vi "Analy Json.vi"(8 "error in (no error)":errorcluster, 10 "body":string="{\"error_code\":0,\"error_msg\":\"SUCCESS\",\"log_id\":3501517038,\"timestamp\":1684306701,\"cached\":0,\"result\":{\"face_num\":7,\"face_list\":[{\"face_token\":\"9dc85bb57dba77ceee2717260b4e6c8a\",\"location\":{\"left\":515.27,\"top\":41.56,\"width\":29,\"height\":31,\"rotation\":13},\"face_probability\":1,\"angle\":{\"yaw\":21.28,\"pitch\":5.54,\"roll\":10.68}},{\"face_token\":\"519822cd005f9fd56a774038260bf9c1\",\"location\":{\"left\":242.84,\"top\":19.73,\"width\":29,\"height\":29,\"rotation\":33},\"face_probability\":1,\"angle\":{\"yaw\":-2.53,\"pitch\":12.63,\"roll\":30.73}},{\"face_token\":\"0cb54c44f353f8f4b24468424f908c8a\",\"location\":{\"left\":150.92,\"top\":30.76,\"width\":30,\"height\":28,\"rotation\":6},\"face_probability\":0.99,\"angle\":{\"yaw\":-1.15,\"pitch\":9.32,\"roll\":2.81}},{\"face_token\":\"8612e393bdc06ac7a96a46a15dd12818\",\"location\":{\"left\":367.55,\"top\":29.17,\"width\":27,\"height\":31,\"rotation\":9},\"face_probability\":1,\"angle\":{\"yaw\":-14.5,\"pitch\":3.18,\"roll\":7.23}},{\"face_token\":\"1f123ecde6098c6bc67fbb6ddb0b806a\",\"location\":{\"left\":447,\"top\":38.09,\"width\":29,\"height\":27,\"rotation\":10},\"face_probability\":1,\"angle\":{\"yaw\":-8.18,\"pitch\":8.23,\"roll\":10.84}},{\"face_token\":\"b994523fe7b95fddfed7fbed407f0b6f\",\"location\":{\"left\":80.83,\"top\":43.37,\"width\":30,\"height\":26,\"rotation\":23},\"face_probability\":1,\"angle\":{\"yaw\":-14.98,\"pitch\":12.31,\"roll\":24.44}},{\"face_token\":\"da3ec671683a7d13f9daffcd54db10f0\",\"location\":{\"left\":300.6,\"top\":29.25,\"width\":28,\"height\":27,\"rotation\":9},\"face_probability\":1,\"angle\":{\"yaw\":-7.29,\"pitch\":8.2,\"roll\":7.41}}]}}" caption="体部") -> (0 "error out":errorcluster, 2 "face_list":T3[](array[typedef]), 3 "All info":T1)   [LabVIEW 2025]
uses:
  controls/face_list.ctl
  controls/All info.ctl
  controls/Return Info.ctl
  <vilib>/addons/_JKI.lib/Serialization/JSON/JKI JSON Serialization.lvlib
  <vilib>/Utility/Data Type/NI_Data Type.lvlib
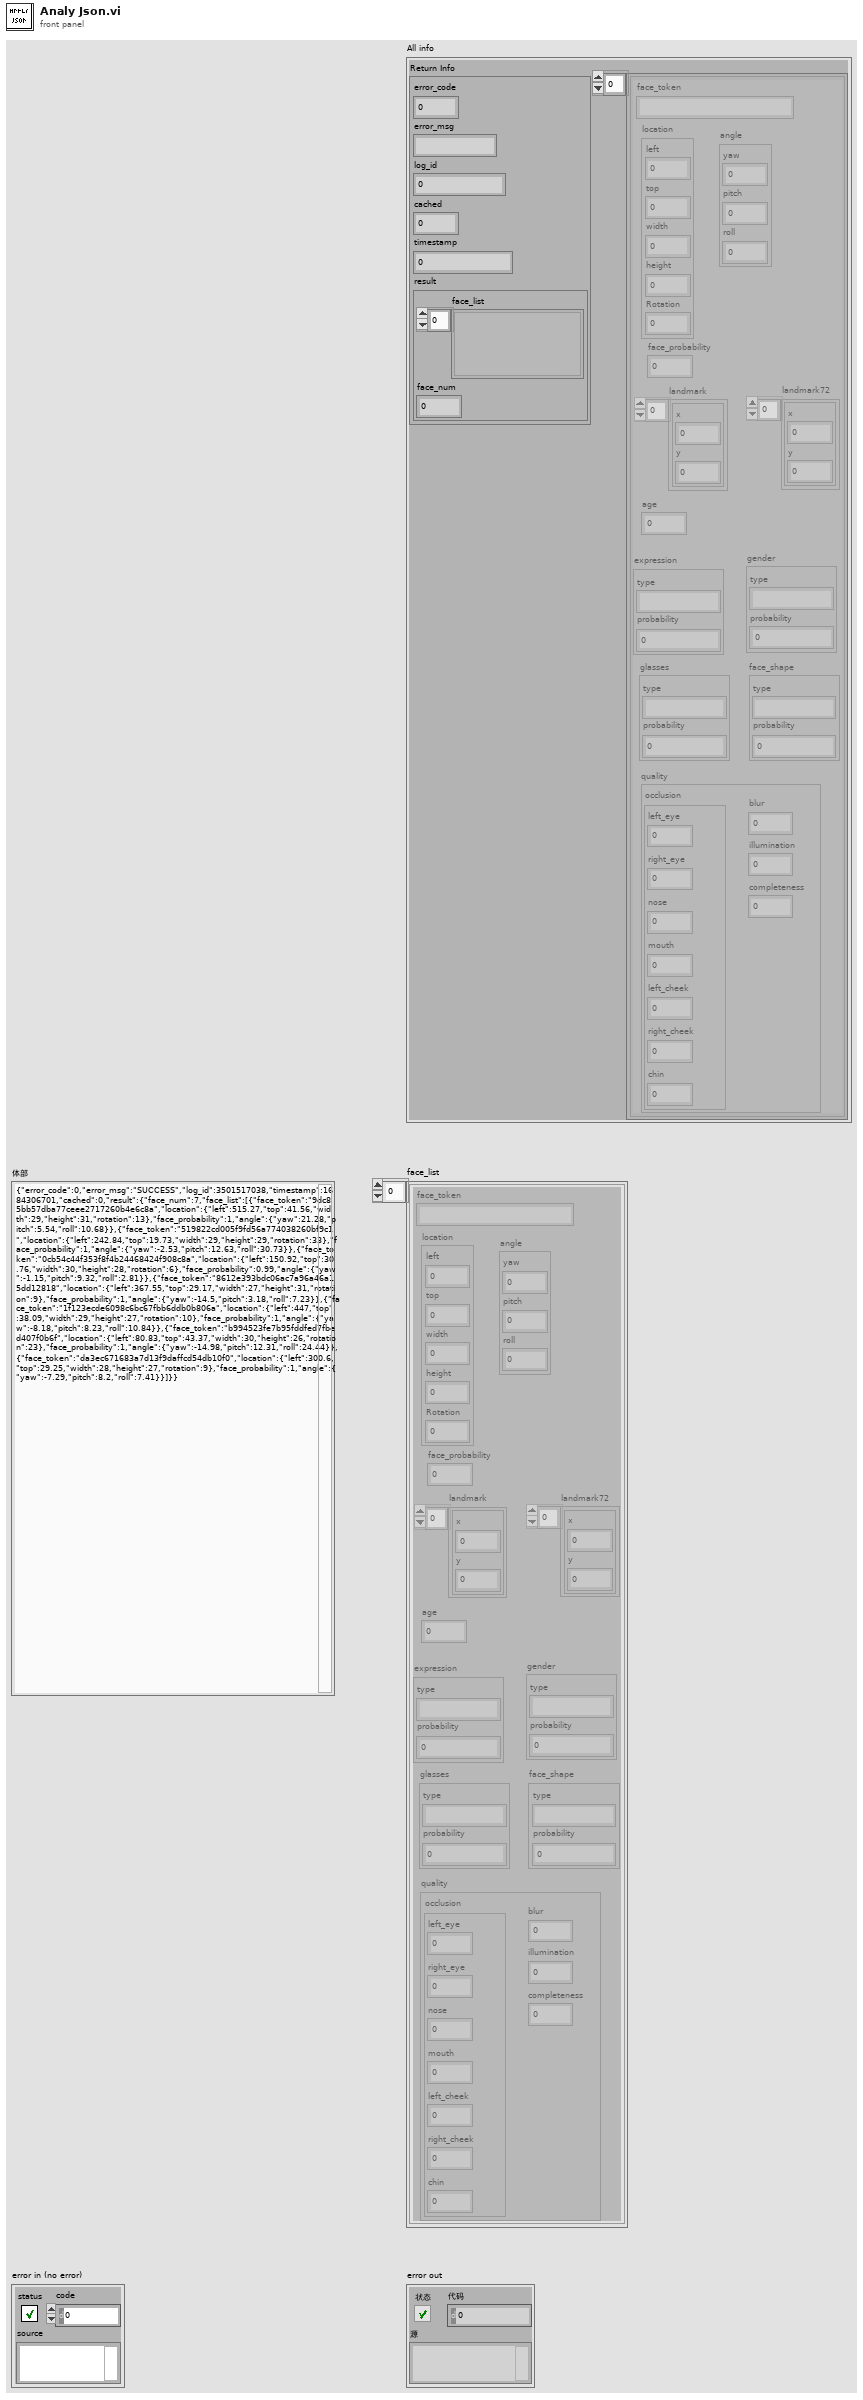
[diagram p1: front panel]
types:
  T1 = typedef "All info.ctl" = cluster{"Return Info":T2, T3[]}
  T2 = typedef "Return Info.ctl" = cluster{"error_code":i32, "error_msg":string, "log_id":u64, "cached":u64, "timestamp":u64, "result":cluster{"face_list":variant[], "face_num":i32}}
  T3 = typedef "face_list.ctl" = cluster{"location":cluster{"left":i32, "top":i32, "width":i32, "height":i32, "Rotation":i32}, "face_probability":dbl, "age":dbl, "landmark":cluster{"x":u32, "y":u32}[], "landmark72":cluster{"x":u32, "y":u32}[], "angle":cluster{"yaw":dbl, "pitch":dbl, "roll":dbl}, "face_token":string, "face_shape":cluster{"type":string, "probability":dbl}, "glasses":cluster{"type":string, "probability":dbl}, "expression":cluster{"type":string, "probability":dbl}, "gender":cluster{"type":string, "probability":dbl}, "quality":cluster{"illumination":i32, "completeness":i32, "blur":i32, "occlusion":cluster{"left_eye":dbl, "right_eye":dbl, "nose":dbl, "mouth":dbl, "left_cheek":dbl, "right_cheek":dbl, "chin":dbl}}}
  T4 = cluster{"left":i32, "top":i32, "width":i32, "height":i32, "Rotation":i32}
  T5 = cluster{"left_eye":dbl, "right_eye":dbl, "nose":dbl, "mouth":dbl, "left_cheek":dbl, "right_cheek":dbl, "chin":dbl}
  T6 = cluster{"occlusion":variant[], "blur":i32, "illumination":i32, "completeness":i32}
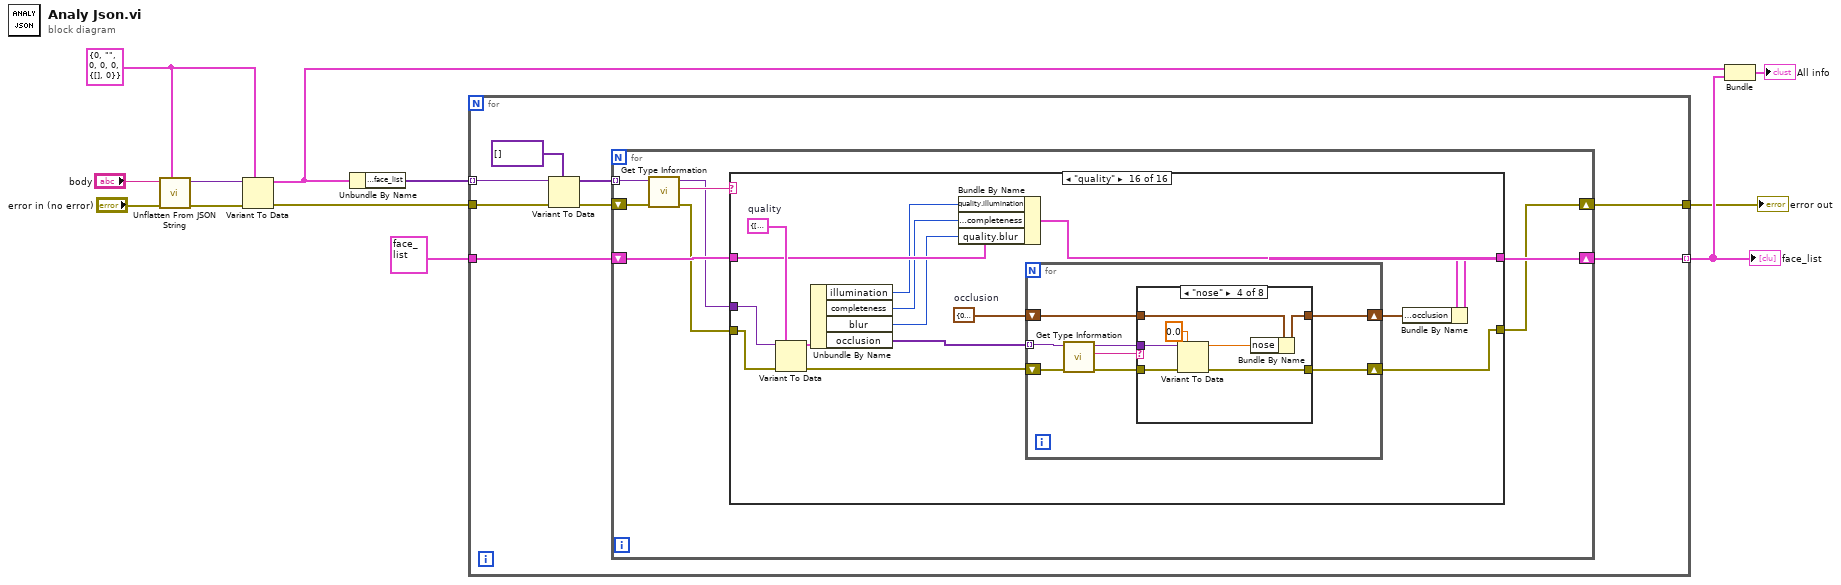
[diagram p0: block diagram]
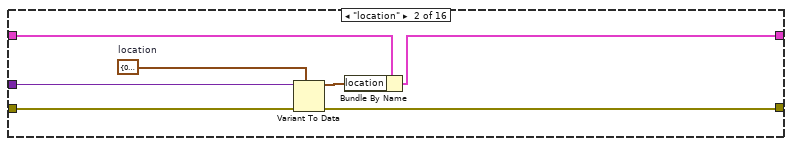
[diagram p3: hidden frame]
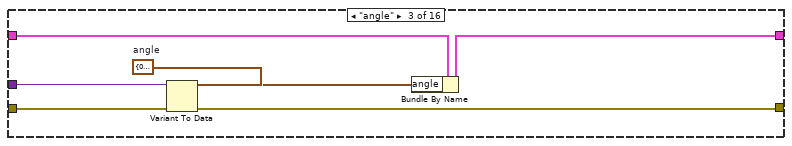
[diagram p4: hidden frame]
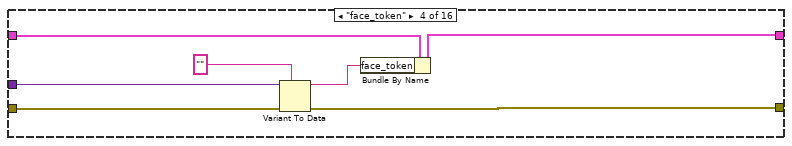
[diagram p5: hidden frame]
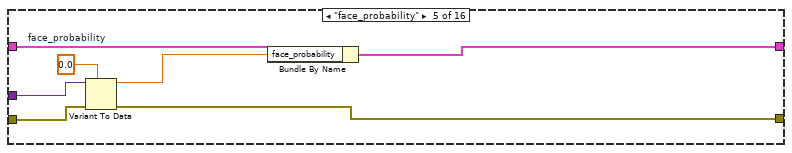
[diagram p6: hidden frame]
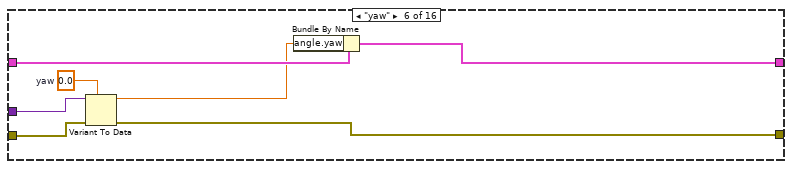
[diagram p7: hidden frame]
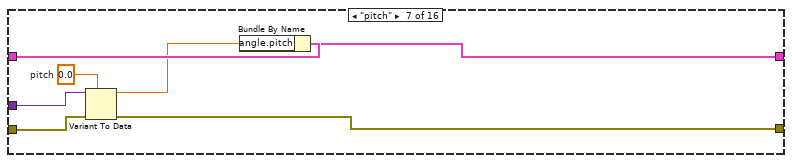
[diagram p8: hidden frame]
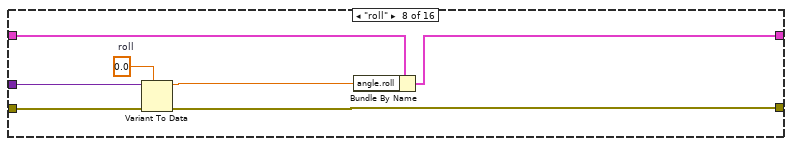
[diagram p9: hidden frame]
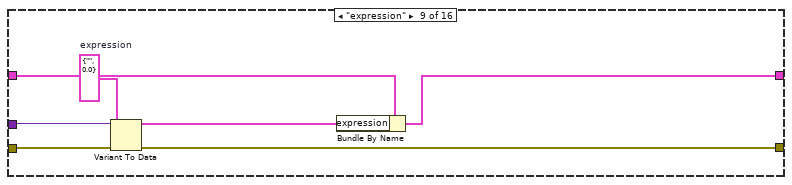
[diagram p10: hidden frame]
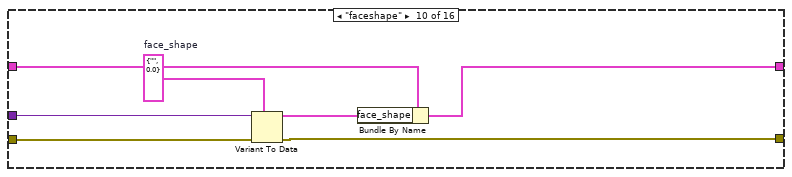
[diagram p11: hidden frame]
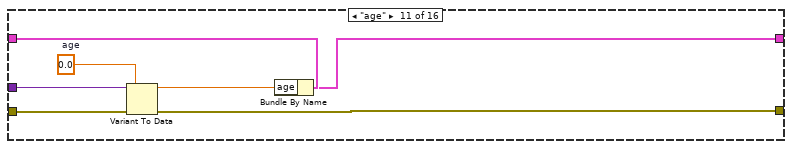
[diagram p12: hidden frame]
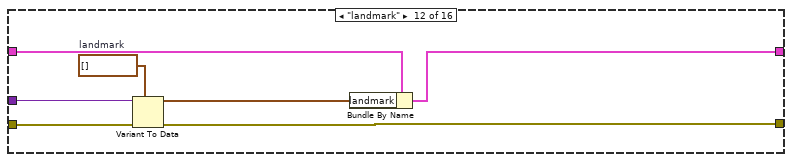
[diagram p13: hidden frame]
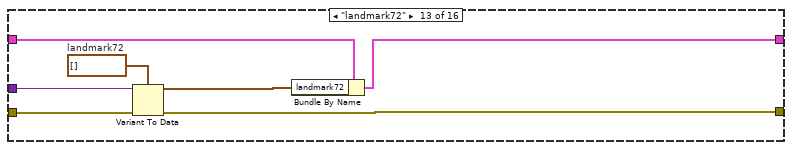
[diagram p14: hidden frame]
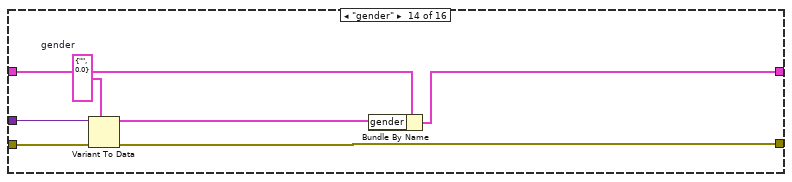
[diagram p15: hidden frame]
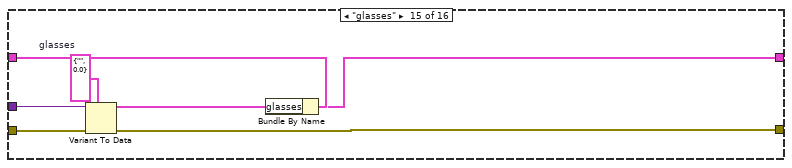
[diagram p16: hidden frame]
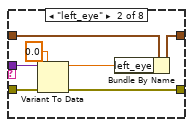
[diagram p18: hidden frame]
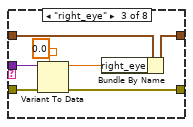
[diagram p19: hidden frame]
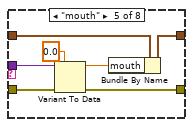
[diagram p20: hidden frame]
diagram:
  w10 = T2 {"error_code"=0, "error_msg"="", "log_id"=0, "cached"=0, "timestamp"=0, "result"={"face_list"=[], "face_num"=0}} ("11")
  n1 = call <vilib>:"Unflatten From JSON String.vi"("Type and Defaults"=w10, "error in"="error in (no error)", "JSON String"="body") -> ("error out"=w12:errorcluster, "Variant"=w11:variant)  [unwired: 7 in]
  n2 = Variant To Data(error in=w12, type=w10, Variant=w11) -> (data=w7:T2, error out=w4:errorcluster)
  n3 = Unbundle By Name(w7) -> ("result.face_list"=w8:variant[])
  n4 = for {
    tunnel: T3 {"location"={"left"=0, "top"=0, "width"=0, "height"=0, "Rotation"=0}, "face_probability"=0.0, "age"=0.0, "landmark"=[], "landmark72"=[], "angle"={"yaw"=0.0, "pitch"=0.0, "roll"=0.0}, "face_token"="", "face_shape"={"type"="", "probability"=0.0}, "glasses"={"type"="", "probability"=0.0}, "expression"={"type"="", "probability"=0.0}, "gender"={"type"="", "probability"=0.0}, "quality"={"illumination"=0, "completeness"=0, "blur"=0, "occlusion"={"left_eye"=0.0, "right_eye"=0.0, "nose"=0.0, "mouth"=0.0, "left_cheek"=0.0, "right_cheek"=0.0, "chin"=0.0}}} -> [w18]
    tunnel: [w17] -> w6 mode=indexing
    tunnel: w8 -> [w16] mode=indexing
    tunnel: w4 -> [w14]
    tunnel: [w13] -> w2
    n5 = Variant To Data(error in=w14, type=variant[] [] ("类型"), Variant=w16) -> (data=w19:variant[], error out=w15:errorcluster)
    n6 = for {
      tunnel: w19 -> [w25] mode=indexing
      shift-right: [w23] -> w17
      shift-left: w18 -> [w27]
      shift-right: [w21] -> w13
      shift-left: w15 -> [w22]
      n7 = call <vilib>:"Get Type Information.vi"("error in (no error)"=w22, "variant"=w25) -> ("error out"=w24:errorcluster, "name"=w26:string)  [unwired: 5 in, 3 out]
      n8 = case shown="\"quality\"" w26 {
        tunnel: w25 -> [_ w36 w38 w48 w57 w64 w71 w78 w80 w92 w99 w106 w113 w120 w127 w141]
        tunnel: w27 -> [w29 w35 w43 w50 w55 w62 w69 w76 w85 w91 w97 w104 w111 w119 w126 w134]
        tunnel: [w29 w33 w42 w49 w53 w60 w67 w72 w84 w88 w93 w100 w109 w116 w123 w133] -> w23
        tunnel: w24 -> [w28 w31 w39 w47 w52 w59 w66 w74 w83 w90 w95 w102 w107 w118 w125 w136]
        tunnel: [w28 w32 w37 w44 w51 w58 w65 w73 w79 w89 w94 w101 w108 w117 w124 w142] -> w21
        frame "", Default {
        }
        frame "location" {
          w30 = T4 {"left"=0, "top"=0, "width"=0, "height"=0, "Rotation"=0}  # location
          n9 = Variant To Data(error in=w31, type=w30, Variant=w36) -> (data=w34:T4, error out=w32:errorcluster)
          n10 = Bundle By Name(cluster=w35, "location"=w34) -> (w33:T3)
        }
        frame "angle" {
          w41 = cluster{"yaw":dbl, "pitch":dbl, "roll":dbl} {"yaw"=0.0, "pitch"=0.0, "roll"=0.0}  # angle
          n11 = Variant To Data(error in=w39, type=w41, Variant=w38) -> (data=w40:cluster{"yaw":dbl, "pitch":dbl, "roll":dbl}, error out=w37:errorcluster)
          n12 = Bundle By Name(cluster=w43, "angle"=w40) -> (w42:T3)
        }
        frame "face_token" {
          n13 = Variant To Data(error in=w47, type="" ("face_token"), Variant=w48) -> (data=w45:string, error out=w44:errorcluster)
          n14 = Bundle By Name(cluster=w50, "face_token"=w45) -> (w49:T3)
        }
        frame "face_probability" {
          w56 = 0.0  # face_probability
          n15 = Variant To Data(error in=w52, type=w56, Variant=w57) -> (data=w54:dbl, error out=w51:errorcluster)
          n16 = Bundle By Name(cluster=w55, "face_probability"=w54) -> (w53:T3)
        }
        frame "yaw" {
          w63 = 0.0  # yaw
          n17 = Variant To Data(error in=w59, type=w63, Variant=w64) -> (data=w61:dbl, error out=w58:errorcluster)
          n18 = Bundle By Name(cluster=w62, "angle.yaw"=w61) -> (w60:T3)
        }
        frame "pitch" {
          w70 = 0.0  # pitch
          n19 = Variant To Data(error in=w66, type=w70, Variant=w71) -> (data=w68:dbl, error out=w65:errorcluster)
          n20 = Bundle By Name(cluster=w69, "angle.pitch"=w68) -> (w67:T3)
        }
        frame "roll" {
          w77 = 0.0  # roll
          n21 = Variant To Data(error in=w74, type=w77, Variant=w78) -> (data=w75:dbl, error out=w73:errorcluster)
          n22 = Bundle By Name(cluster=w76, "angle.roll"=w75) -> (w72:T3)
        }
        frame "expression" {
          w81 = cluster{"type":string, "probability":sgl} {"type"="", "probability"=0.0}  # expression
          n23 = Variant To Data(error in=w83, type=w81, Variant=w80) -> (data=w82:cluster{"type":string, "probability":sgl}, error out=w79:errorcluster)
          n24 = Bundle By Name(cluster=w85, "expression"=w82) -> (w84:T3)
        }
        frame "faceshape" {
          w86 = cluster{"type":string, "probability":dbl} {"type"="", "probability"=0.0}  # face_shape
          n25 = Variant To Data(error in=w90, type=w86, Variant=w92) -> (data=w87:cluster{"type":string, "probability":dbl}, error out=w89:errorcluster)
          n26 = Bundle By Name(cluster=w91, "face_shape"=w87) -> (w88:T3)
        }
        frame "age" {
          w98 = 0.0  # age
          n27 = Variant To Data(error in=w95, type=w98, Variant=w99) -> (data=w96:dbl, error out=w94:errorcluster)
          n28 = Bundle By Name(cluster=w97, "age"=w96) -> (w93:T3)
        }
        frame "landmark" {
          w105 = cluster{"x":u32, "y":u32}[] []  # landmark
          n29 = Variant To Data(error in=w102, type=w105, Variant=w106) -> (data=w103:cluster{"x":u32, "y":u32}[], error out=w101:errorcluster)
          n30 = Bundle By Name(cluster=w104, "landmark"=w103) -> (w100:T3)
        }
        frame "landmark72" {
          w112 = cluster{"x":u32, "y":u32}[] []  # landmark72
          n31 = Variant To Data(error in=w107, type=w112, Variant=w113) -> (data=w110:cluster{"x":u32, "y":u32}[], error out=w108:errorcluster)
          n32 = Bundle By Name(cluster=w111, "landmark72"=w110) -> (w109:T3)
        }
        frame "gender" {
          w114 = cluster{"type":string, "probability":dbl} {"type"="", "probability"=0.0}  # gender
          n33 = Variant To Data(error in=w118, type=w114, Variant=w120) -> (data=w115:cluster{"type":string, "probability":dbl}, error out=w117:errorcluster)
          n34 = Bundle By Name(cluster=w119, "gender"=w115) -> (w116:T3)
        }
        frame "glasses" {
          w121 = cluster{"type":string, "probability":dbl} {"type"="", "probability"=0.0}  # glasses
          n35 = Variant To Data(error in=w125, type=w121, Variant=w127) -> (data=w122:cluster{"type":string, "probability":dbl}, error out=w124:errorcluster)
          n36 = Bundle By Name(cluster=w126, "glasses"=w122) -> (w123:T3)
        }
        frame "quality" {
          w135 = T5 {"left_eye"=0.0, "right_eye"=0.0, "nose"=0.0, "mouth"=0.0, "left_cheek"=0.0, "right_cheek"=0.0, "chin"=0.0}  # occlusion
          w140 = T6 {"occlusion"=[], "blur"=0, "illumination"=0, "completeness"=0}  # quality
          n37 = Variant To Data(error in=w136, type=w140, Variant=w141) -> (data=w139:T6, error out=w137:errorcluster)
          n38 = Unbundle By Name(w139) -> ("illumination"=w130:i32, "completeness"=w129:i32, "blur"=w128:i32, "occlusion"=w138:variant[])
          n39 = Bundle By Name(cluster=w134, "quality.illumination"=w130, "quality.completeness"=w129, "quality.blur"=w128) -> (w131:T3)
          n40 = for {
            shift-right: [w146] -> w142
            shift-left: w137 -> [w148]
            tunnel: w138 -> [w143] mode=indexing
            shift-right: [w144] -> w132
            shift-left: w135 -> [w145]
            n41 = call <vilib>:"Get Type Information.vi"("error in (no error)"=w148, "variant"=w143) -> ("error out"=w147:errorcluster, "name"=w149:string)  [unwired: 5 in, 3 out]
            n42 = case shown="\"nose\"" w149 {
              tunnel: w147 -> [w151 w153 w163 w169 w176 w185 w191 w200]
              tunnel: [w151 w152 w162 w168 w175 w184 w190 w194] -> w146
              tunnel: w145 -> [w150 w155 w161 w172 w179 w182 w189 w199]
              tunnel: [w150 w154 w160 w167 w174 w181 w188 w198] -> w144
              tunnel: w143 -> [_ w156 w159 w170 w177 w183 w192 w196]
              frame "", Default {
              }
              frame "left_eye" {
                n43 = Variant To Data(error in=w153, type=0.0, Variant=w156) -> (data=w158:dbl, error out=w152:errorcluster)
                n44 = Bundle By Name(cluster=w155, "left_eye"=w158) -> (w154:T5)
              }
              frame "right_eye" {
                n45 = Variant To Data(error in=w163, type=0.0, Variant=w159) -> (data=w165:dbl, error out=w162:errorcluster)
                n46 = Bundle By Name(cluster=w161, "right_eye"=w165) -> (w160:T5)
              }
              frame "nose" {
                n47 = Variant To Data(error in=w169, type=0.0, Variant=w170) -> (data=w166:dbl, error out=w168:errorcluster)
                n48 = Bundle By Name(cluster=w172, "nose"=w166) -> (w167:T5)
              }
              frame "mouth" {
                n49 = Variant To Data(error in=w176, type=0.0, Variant=w177) -> (data=w173:dbl, error out=w175:errorcluster)
                n50 = Bundle By Name(cluster=w179, "mouth"=w173) -> (w174:T5)
              }
              frame "left_cheek" {
                n51 = Variant To Data(error in=w185, type=0.0, Variant=w183) -> (data=w180:dbl, error out=w184:errorcluster)
                n52 = Bundle By Name(cluster=w182, "left_cheek"=w180) -> (w181:T5)
              }
              frame "right_cheek" {
                n53 = Variant To Data(error in=w191, type=0.0, Variant=w192) -> (data=w187:dbl, error out=w190:errorcluster)
                n54 = Bundle By Name(cluster=w189, "right_cheek"=w187) -> (w188:T5)
              }
              frame "chin" {
                n55 = Variant To Data(error in=w200, type=0.0, Variant=w196) -> (data=w197:dbl, error out=w194:errorcluster)
                n56 = Bundle By Name(cluster=w199, "chin"=w197) -> (w198:T5)
              }
            }
          }
          n57 = Bundle By Name(cluster=w131, "quality.occlusion"=w132) -> (w133:T3)
        }
      }
    }
  }
  "face_list" <- w6
  "error out" <- w2
  n58 = Bundle("11"=w7, w6) -> (→"All info":cluster{"11":T2, T3[]})  [unwired: 1 in]
